vi "PXI-Create Device Maps.vi"(0 "Num AO":i32[](array[numeric]), 5 "Num AI":i32[](array[numeric]), 7 "Slot Num":u32[](array[numeric]), 11 "error in (no error)":errorcluster) -> (4 "AO Map":T1, 6 "AI Map":T1, 15 "error out":errorcluster)   [LabVIEW 2020]
panel:
  out "AI Phys Dev to DAQ Chan":i32[][](array[numeric])
  out "AI DAQ Chan to Phys Dev":i32[][](array[numeric])
  out "AO Phys Dev to DAQ Chan":i32[][](array[numeric])
  out "AO DAQ Chan to Phys Dev":i32[][](array[numeric])
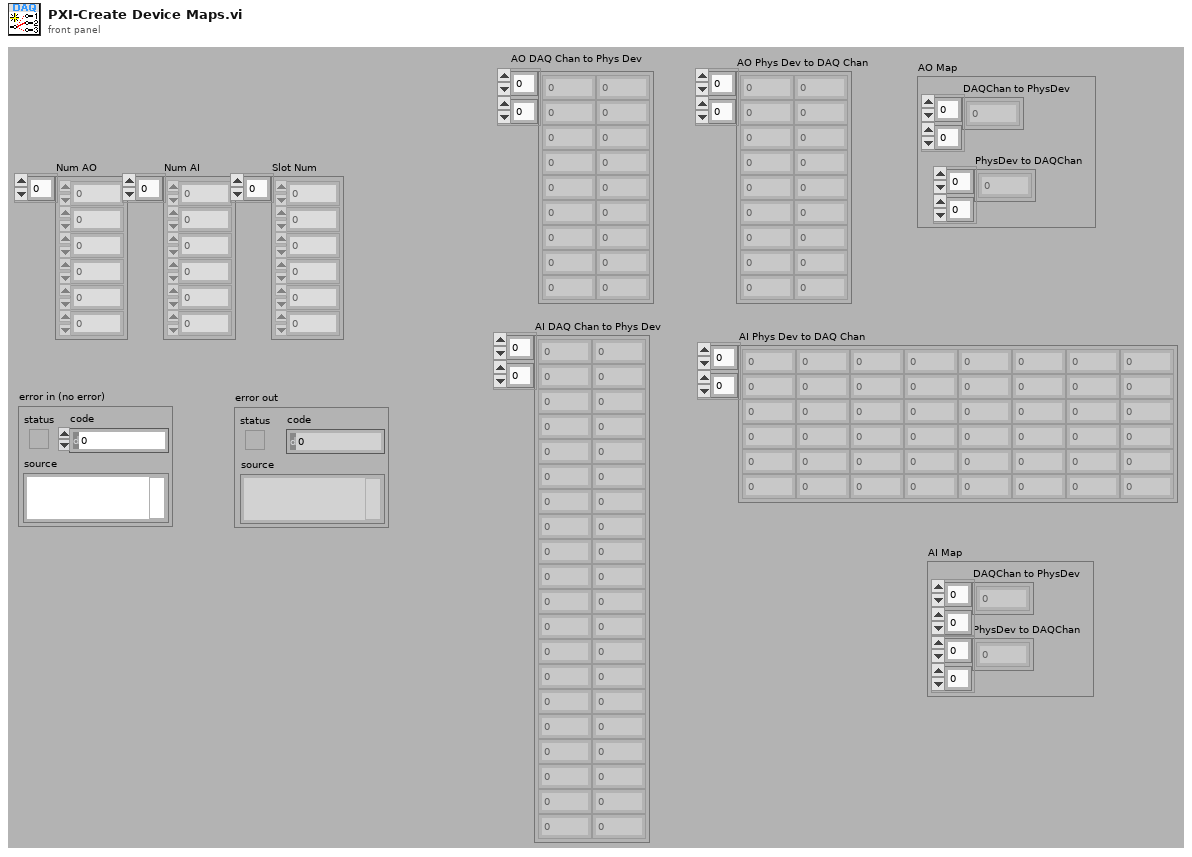
[diagram p1: front panel]
types:
  T1 = cluster{"DAQChan to PhysDev":i32[][], "PhysDev to DAQChan":i32[][]}
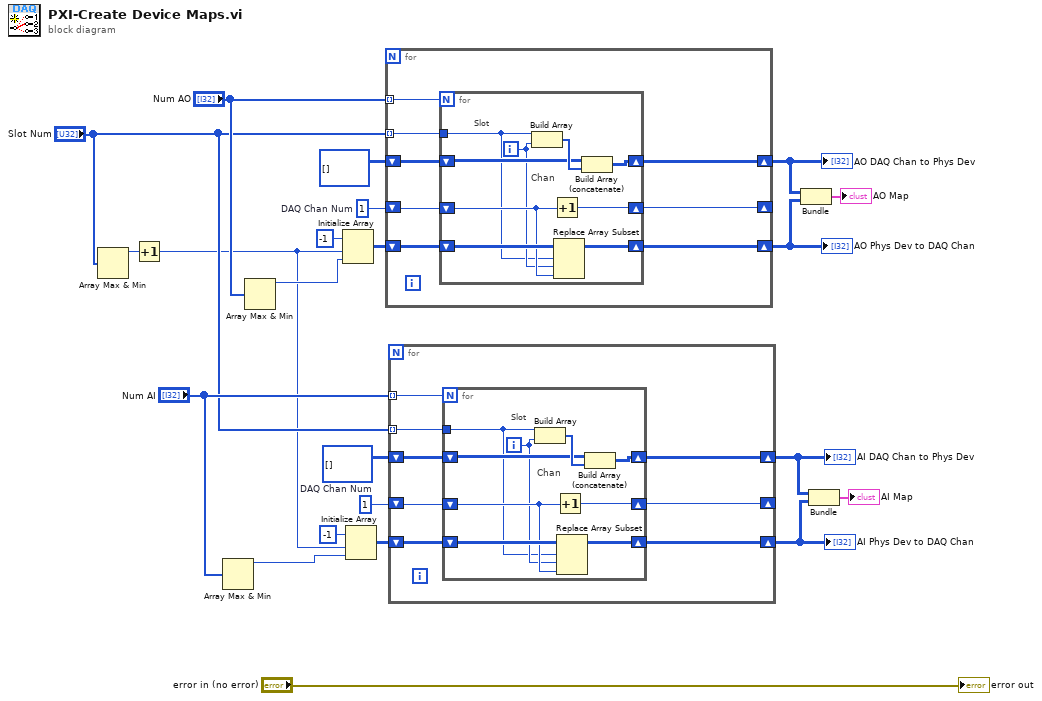
[diagram p0: block diagram]
diagram:
  w17 = 1  # DAQ Chan Num
  w21 = 1  # DAQ Chan Num
  n1 = Array Max & Min(array="Slot Num") -> (max value=w2:u32)  [unwired: 3 out]
  n2 = Increment(x=w2) -> (x+1=w1:u32)
  n3 = Array Max & Min(array="Num AI") -> (max value=w14:i32)  [unwired: 3 out]
  n4 = Array Max & Min(array="Num AO") -> (max value=w11:i32)  [unwired: 3 out]
  n5 = Initialize Array(-1 ("element"), w1, w11) -> (w19:i32[][])
  n6 = Initialize Array(-1 ("element"), w1, w14) -> (w15:i32[][])
  n7 = for {
    tunnel: "Num AO" -> [w30] mode=indexing
    shift-right: [w26] -> w10
    shift-left: i32[][] [] -> [w29]
    shift-right: [w27] -> _
    shift-left: w21 -> [w28]
    shift-right: [w24] -> w9
    shift-left: w19 -> [w25]
    tunnel: "Slot Num" -> [w23] mode=indexing
    n8 = for {
      N: w30 -> [_]
      shift-right: [w38] -> w26
      shift-left: w29 -> [w36]
      shift-right: [w39] -> w27
      shift-left: w28 -> [w33]
      shift-right: [w34] -> w24
      shift-left: w25 -> [w35]
      tunnel: w23 -> [w31]
      i -> [w32]
      # "Chan"
      # "Slot"
      n9 = Build Array(w31, w32) -> (w37:u32[])
      n10 = Increment(x=w33) -> (x+1=w39:i32)
      n11 = Replace Array Subset(array=w35, new element=w33, index (row)=w31, index (col)=w32) -> (w34:i32[][])
      n12 = Build Array (concatenate)(w36, w37) -> (w38:u32[][])
    }
  }
  "AO DAQ Chan to Phys Dev" <- w10
  "AO Phys Dev to DAQ Chan" <- w9
  n13 = for {
    tunnel: "Num AI" -> [w47] mode=indexing
    shift-right: [w43] -> w7
    shift-left: i32[][] [] -> [w46]
    shift-right: [w44] -> _
    shift-left: w17 -> [w45]
    shift-right: [w41] -> w6
    shift-left: w15 -> [w42]
    tunnel: "Slot Num" -> [w40] mode=indexing
    n14 = for {
      N: w47 -> [_]
      shift-right: [w55] -> w43
      shift-left: w46 -> [w53]
      shift-right: [w56] -> w44
      shift-left: w45 -> [w50]
      shift-right: [w51] -> w41
      shift-left: w42 -> [w52]
      tunnel: w40 -> [w48]
      i -> [w49]
      # "Chan"
      # "Slot"
      n15 = Build Array(w48, w49) -> (w54:u32[])
      n16 = Increment(x=w50) -> (x+1=w56:i32)
      n17 = Replace Array Subset(array=w52, new element=w50, index (row)=w48, index (col)=w49) -> (w51:i32[][])
      n18 = Build Array (concatenate)(w53, w54) -> (w55:u32[][])
    }
  }
  "AI DAQ Chan to Phys Dev" <- w7
  "AI Phys Dev to DAQ Chan" <- w6
  n19 = Bundle(w10, w9) -> (→"AO Map":cluster{u32[][], i32[][]})  [unwired: 1 in]
  n20 = Bundle(w7, w6) -> (→"AI Map":cluster{u32[][], i32[][]})  [unwired: 1 in]
  "error out" <- "error in (no error)"
